vi "32xx_Lect_U_I.vi"(8 "error in (no error)":errorcluster, 10 "Select Voie":i32(ring)=1 items=["CH 1"=1, "CH 2"=2, "CH 3"=3], 11 "VISA resource name":refnum<visa-resource-name>="COM3") -> (0 "error out":errorcluster, 3 "VISA resource name out":refnum<visa-resource-name>="COM3")   [LabVIEW 2020]
doc: "Configures the power supply's output voltage level, channel, voltage range, and enables or disables the output."
panel:
  out "ON/OFF":T1=enum."ON"
  out "Local/Remote":enum16{"Local", "Remote"}(ring)=enum."Remote"
  out "Sortie (V/A)":dbl=2.5
  in  "Produit":T2(ring)
  in  "Chaîne\nSelect.\nParam.":string(combo)="VOLT" caption="Select. Param."
  # "© 2020 elc ALL RIGHTS RESERVED"
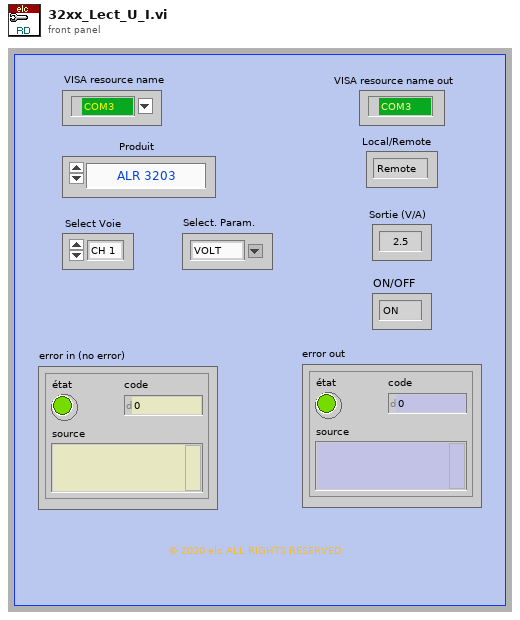
[diagram p1: front panel]
types:
  T1 = typedef "32xx_Enum_ON_OFF.ctl" = enum16{"OFF", "ON"}
  T2 = enum16{"ALR 3203", "ALR 3220", "ALR 3206D", "ALR 3206T"}
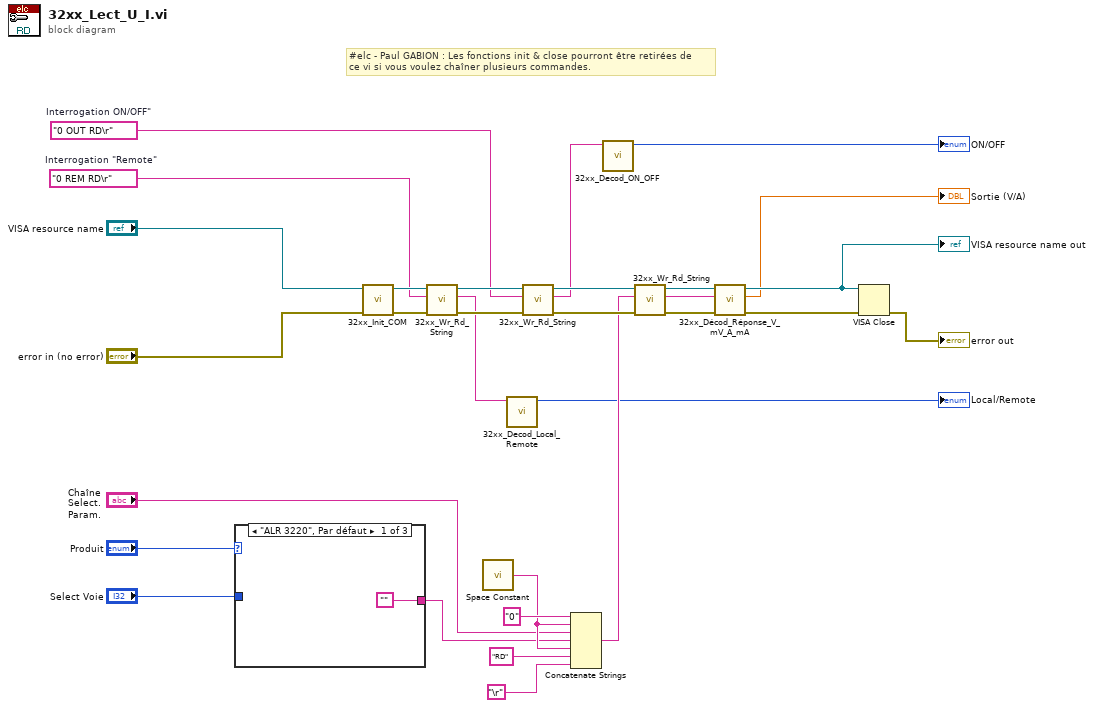
[diagram p0: block diagram]
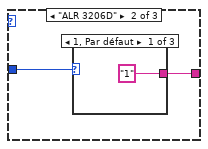
[diagram p2: hidden frame]
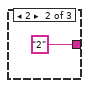
[diagram p3: hidden frame]
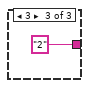
[diagram p4: hidden frame]
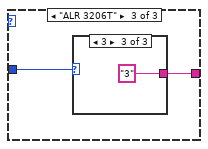
[diagram p5: hidden frame]
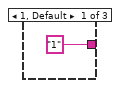
[diagram p6: hidden frame]
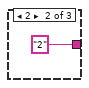
[diagram p7: hidden frame]
diagram:
  w22 = "0 OUT RD\r"  # Interrogation ON/OFF"
  w25 = "0 REM RD\r"  # Interrogation "Remote"
  # "#elc - Paul GABION : Les fonctions init & close pourront être retirées de\nce vi si vous voulez chaîner plusieurs commandes."
  n1 = case shown="\"ALR 3220\", Par défaut" "Produit" {
    tunnel: "Select Voie" -> [_ w33 w38]
    tunnel: ["" w32 w37] -> w15
    frame "ALR 3220", Default {
    }
    frame "ALR 3206D" {
      n2 = case shown="1, Par défaut" w33 {
        tunnel: ["1" ("chaîne") "2" ("chaîne") "2" ("chaîne")] -> w32
        frame 1, Default {
        }
        frame 2 {
        }
        frame 3 {
        }
      }
    }
    frame "ALR 3206T" {
      n3 = case shown="3" w38 {
        tunnel: ["1" ("chaîne") "2" ("chaîne") "3" ("chaîne")] -> w37
        frame 1, Default {
        }
        frame 2 {
        }
        frame 3 {
        }
      }
    }
  }
  n4 = call "32xx_Init_COM.vi"("Entrée d'erreur"="error in (no error)", "Port d'entrée"="VISA resource name") -> ("Sortie d'erreur"=w26:errorcluster, "Port de sortie"=w27:refnum<visa-resource-name>)  [unwired: 7 in, 1 out]
  n5 = call "32xx_Wr_Rd_String.vi"("entrée d'erreur"=w26, "String In"=w25, "Visa In"=w27) -> ("sortie d'erreur"=w23:errorcluster, "Réponse"=w4:string, "Visa Out"=w24:refnum<visa-resource-name>)  [unwired: 4 in, 2 out]
  n6 = call <vilib>:"Space Constant.vi"() -> ("String"=w17:string)
  n7 = call "32xx_Decod_Local_Remote.vi"("Réponse"=w4) -> ("Local/Remote"=→"Local/Remote":enum16{"Local", "Remote"})  [unwired: 10 in]
  n8 = call "32xx_Wr_Rd_String.vi"("entrée d'erreur"=w23, "String In"=w22, "Visa In"=w24) -> ("sortie d'erreur"=w20:errorcluster, "Réponse"=w2:string, "Visa Out"=w21:refnum<visa-resource-name>)  [unwired: 4 in, 2 out]
  n9 = Concatenate Strings("0" ("chaîne"), w17, "Chaîne\nSelect.\nParam.", w15, w17, "RD" ("chaîne"), "\r") -> (w13:string)
  n10 = call "32xx_Decod_ON_OFF.vi"("Réponse"=w2) -> ("ON/OFF"=→"ON/OFF":T1)  [unwired: 10 in]
  n11 = call "32xx_Wr_Rd_String.vi"("entrée d'erreur"=w20, "String In"=w13, "Visa In"=w21) -> ("sortie d'erreur"=w9:errorcluster, "Réponse"=w5:string, "Visa Out"=w10:refnum<visa-resource-name>)  [unwired: 4 in, 2 out]
  n12 = call "32xx_Décod_Réponse_V_mV_A_mA.vi"("entrée d'erreur"=w9, "Chaîne\nd'entrée"=w5, "Visa In"=w10) -> ("sortie d'erreur"=w7:errorcluster, "Sortie (V) / (A)"=→"Sortie (V/A)":dbl, "Visa Out"=w8:refnum<visa-resource-name>)  [unwired: 4 in, 2 out]
  "VISA resource name out" <- w8
  n13 = VISA Close(VISA resource name=w8, error in (no error)=w7) -> (error out=→"error out":errorcluster)
